vi "zad6_write.vi"() -> ()   [LabVIEW 2025]
panel:
  in  "error in":errorcluster
  out "error out":errorcluster
  in  "Array":bool[][][][][][][][][][](array[boolean])
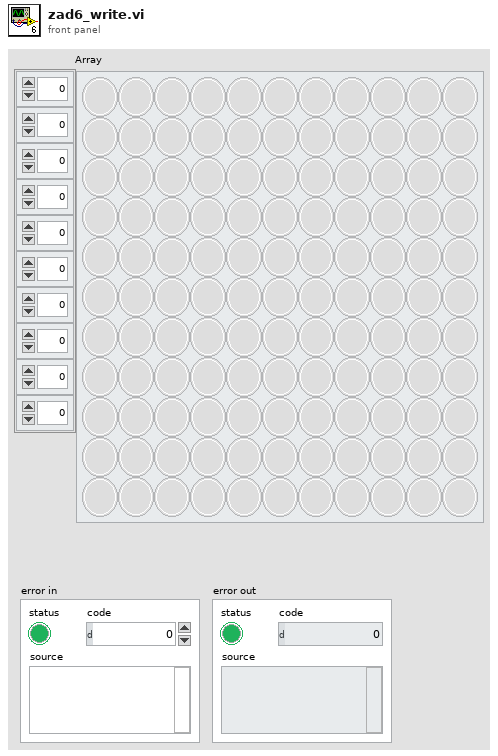
[diagram p1: front panel]
types:
  T1 = enum16{"open", "replace", "create", "open or create", "replace or create", "replace or create with confirmation"}
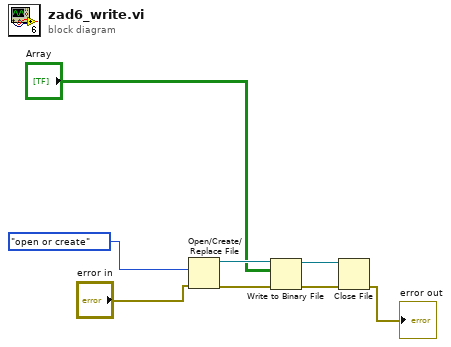
[diagram p0: block diagram]
diagram:
  n1 = Open/Create/Replace File(error in="error in", operation (0:open)=T1."open or create") -> (refnum out=w8:refnum<file>, error out=w4:errorcluster)  [unwired: 4 in, 1 out]
  n2 = Write to Binary File(file (use dialog)=w8, data="Array", error in=w4) -> (refnum out=w7:refnum<file>, error out=w5:errorcluster)  [unwired: 3 in, 1 out]
  n3 = Close File(refnum=w7, error in=w5) -> (error out=→"error out":errorcluster)  [unwired: 1 out]
